vi "GetFrameNames__slk_mt.vi"(8 "error in (no error)":errorcluster, 11 "case model in":refnum<class "CaseModel__slk_mt.lvclass">) -> (0 "error out":errorcluster, 2 "frame names":string[](array[string]), 3 "case model out":refnum<class "CaseModel__slk_mt.lvclass">)   [LabVIEW 2013, in "Lazyboots Menu Tool.lvlib" / "CaseModel__slk_mt.lvclass"]
doc: "Returns all frame names of a case model object."
uses:
  CaseModel__slk_mt.lvclass
panel:
  # "GetFrameNames__slk_mt.vi\nReturns all frame names of a case model object.\n\nNOTICE -- YOU MUST LEAVE THIS NOTICE IN PLACE.\n\nCopyright (c) 2011, LIANG LIU Shawn.Liu.cn@gmail.com\nAll rights reserved.\n\nRedistribution and use in source and binary forms, with or without modification, are permitted provided that the following conditions are met:\n-Redistributions of source code must retain the above copyright notice, this list of conditions and the following disclaimer.\n-Redistributions in binary form must reproduce the above copyright notice, this list of conditions and the following disclaimer in the documentation and/or other materials provided with the distribution.\n-Neither the name of the eLp nor the names of its contributors may be used to endorse or promote products derived from this software without specific prior written permission.\n\nTHIS SOFTWARE IS PROVIDED BY THE COPYRIGHT HOLDERS AND CONTRIBUTORS \"AS IS\" AND ANY EXPRESS OR IMPLIED WARRANTIES, INCLUDING, BUT NOT LIMITED TO, THE IMPLIED WARRANTIES OF MERCHANTABILITY AND FITNESS FOR A PARTICULAR PURPOSE ARE DISCLAIMED. IN NO EVENT SHALL THE COPYRIGHT HOLDER OR CONTRIBUTORS BE LIABLE FOR ANY DIRECT, INDIRECT, INCIDENTAL, SPECIAL, EXEMPLARY, OR CONSEQUENTIAL DAMAGES (INCLUDING, BUT NOT LIMITED TO, PROCUREMENT OF SUBSTITUTE GOODS OR SERVICES; LOSS OF USE, DATA, OR PROFITS; OR BUSINESS INTERRUPTION) HOWEVER CAUSED AND ON ANY THEORY OF LIABILITY, WHETHER IN CONTRACT, STRICT LIABILITY, OR TORT (INCLUDING NEGLIGENCE OR OTHERWISE) ARISING IN ANY WAY OUT OF THE USE OF THIS SOFTWARE, EVEN IF ADVISED OF THE POSSIBILITY OF SUCH DAMAGE."
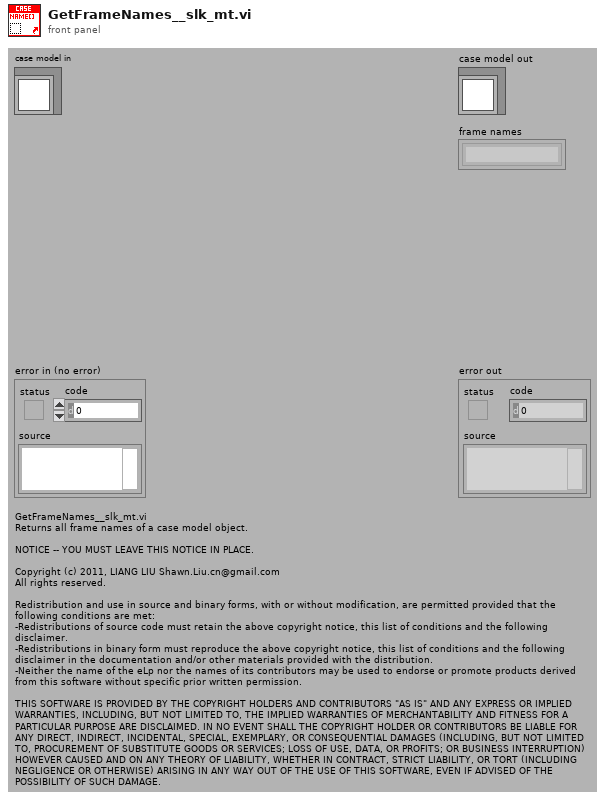
[diagram p1: front panel]
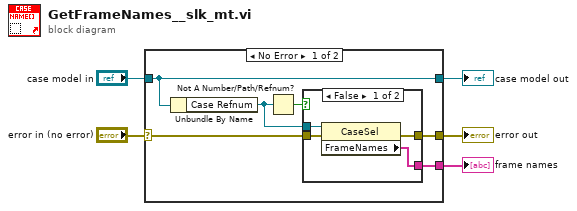
[diagram p0: block diagram]
diagram:
  n1 = case shown="No Error" "error in (no error)" {
    selector: "error in (no error)" -> [w9 w18]
    tunnel: [w8 w18] -> w4
    tunnel: [w11 w17] -> w2
    tunnel: "case model in" -> [w11 w17]
    tunnel: [w10 _] -> w1
    frame No Error {
      n2 = Unbundle By Name(w11) -> ("Case Refnum"=w7:refnum<vi>)
      n3 = Not A Number/Path/Refnum?(number/path/refnum=w7) -> (NaN/Path/Refnum?=w6:bool)
      n4 = case shown="False" w6 {
        tunnel: w7 -> [w15 _]
        tunnel: [w14 _] -> w10
        tunnel: w9 -> [w13 w16]
        tunnel: [w12 w16] -> w8
        frame False {
          n5 = property class="CaseSel"(reference=w15, error in=w13) -> (error out=w12:errorcluster, "FrameNames"=w14:string[])  [unwired: 1 out]
        }
        frame True {
        }
      }
    }
    frame Error {
    }
  }
  "error out" <- w4
  "case model out" <- w2
  "frame names" <- w1
